vi "Interface_GetReference_6x8x6.vi"(0 "reference in":refnum<class>, 5 "error in (no error)":errorcluster) -> (14 "reference out":refnum<class>, 16 "InterfaceOut":refnum<class>, 19 "error out":errorcluster)   [LabVIEW 2016]
doc: "Returns an Interaface that this class implements"
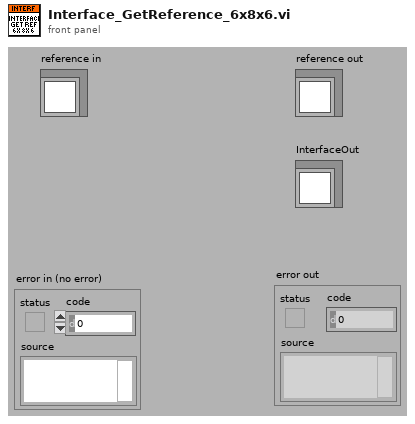
[diagram p1: front panel]
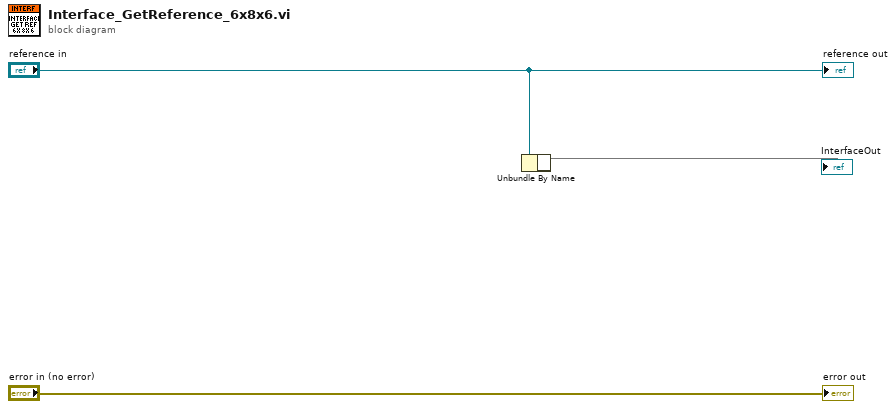
[diagram p0: block diagram]
diagram:
  n1 = Unbundle By Name("reference in") -> (→"InterfaceOut")
  "error out" <- "error in (no error)"
  "reference out" <- "reference in"
